vi "Simulation with Fixed-Point Inputs.vi"() -> ()   [LabVIEW 2023]
doc: "Demonstrates how to simulate the behavior of a fixed-point filter with actual fixed-point inputs."
uses:
  <vilib>/addons/Digital Filter Design/FXPModel.llb/DFD FXP Quantize Coef (Easy).vi
  <vilib>/Utility/VariantDataType/GetNumericFxpInfo.vi
  <vilib>/addons/Digital Filter Design/FXPSim.llb/dfd_Check Input FXP Settings.vi
  <vilib>/addons/Digital Filter Design/FXPSim.llb/dfd_Check SRate Simulation Integer Input.vi
  <vilib>/addons/Digital Filter Design/FXPSim.llb/dfd_FXP Simu.vi
  <vilib>/addons/Digital Filter Design/FXPSim.llb/DFD FXP Postprocessing (I32, 1Ch).vi
  <vilib>/addons/Digital Filter Design/_Objects.llb/DFD Quantization Sources.ctl
  <vilib>/addons/Digital Filter Design/_Objects.llb/DFD FXP Statistics Data.ctl
  <vilib>/addons/Digital Filter Design/FXPSim.llb/SimXnode/DFD FXP Simulation.xnode
  <vilib>/addons/Digital Filter Design/_Objects.llb/DFD Filter Obj.ctl
  <vilib>/addons/Digital Filter Design/_Objects.llb/DFD Filter Coef.ctl
  <vilib>/addons/Digital Filter Design/_Objects.llb/DFD Filter Structure Type Selector.ctl
  <vilib>/addons/Digital Filter Design/_Objects.llb/dfd_Internal Quantization Settings.ctl
  <vilib>/addons/Digital Filter Design/_Objects.llb/dfd_Internal Quantization Srcs.ctl
  <vilib>/addons/Digital Filter Design/_Objects.llb/DFD Coef Norm Type.ctl
  <vilib>/addons/Digital Filter Design/NI_DigFilterLicensed.lvlib
  <vilib>/Analysis/NI_AALBase.lvlib
  <vilib>/addons/Digital Filter Design/NI_DigFilter_FXP.lvlib
  <vilib>/Utility/VariantDataType/VariantType.lvlib
panel:
  out "Filtering Text Report":string
  in  "Output Word Length":i16=16
  out "Error Message":string
  out "Filtering Results":dbl[](graph)
  # "Select Help>>Show Context Help and move the cursor over the VI icon for more information."
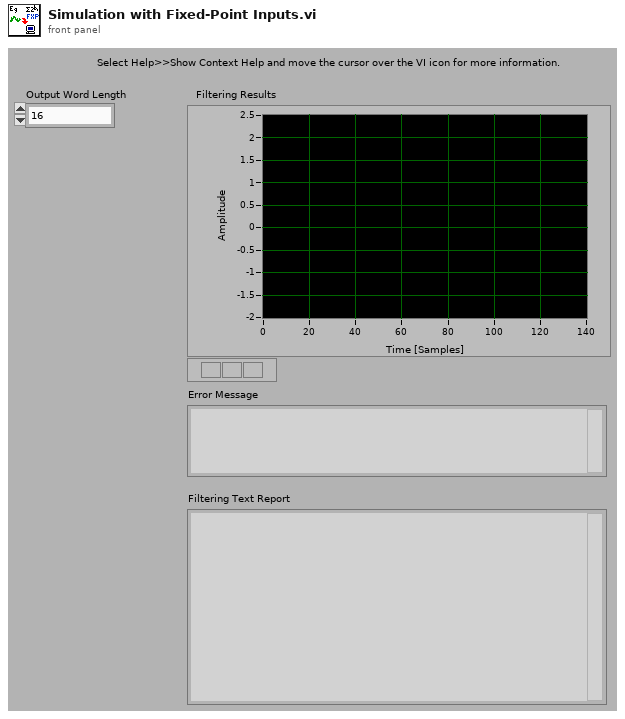
[diagram p1: front panel]
types:
  T1 = enum16{"Butterworth", "Chebyshev", "Inverse Chebyshev", "Elliptic", "Kaiser Window", "Dolph-Chebyshev Window", "Equi-Ripple FIR"}
  T2 = typedef "NI_DigFilterLicensed.lvlib/DFD Filter Obj.ctl" = cluster{"mSRate_Fs":dbl, "mSRate_Version":string, "mSRate_Comments":string, "mSRate_OrgCoef":T3, "mSRate_CurCoef":T3, "mSRate_Quantized?":bool, "mSRate_QCoef":T3, "mSRate_QSettings":T5[], "mSRate_Order":i32, "mSRate_Scaling":cluster{"mSRate_ScaleByPowerOf2?":bool, "mSRate_ScaleType":T7}}
  T3 = typedef "NI_DigFilterLicensed.lvlib/DFD Filter Coef.ctl" = cluster{"type":T4, "gain":dbl, "coef a (k)":dbl[], "coef b (v)":dbl[]}
  T4 = typedef "NI_DigFilterLicensed.lvlib/DFD Filter Structure Type Selector.ctl" = enum16{"Undefined", "FIR Direct Form", "FIR Direct Form Transposed", "FIR Symmetric", "FIR Antisymmetric", "IIR Direct Form I", "IIR Direct Form I Transposed", "IIR Direct Form II", "IIR Direct Form II Transposed", "IIR Cascaded Second Order Sections Form I", "IIR Cascaded Second Order Sections Form I Transposed", "IIR Cascaded Second Order Sections Form II", "IIR Cascaded Second Order Sections Form II Transposed", "Lattice Allpass (basic sections)", "Lattice Allpass (one multiplier sections)", "Lattice Allpass (normalized sections)", "Lattice AR (basic sections)", "Lattice AR (one multiplier sections)", "Lattice AR (normalized sections)", "Lattice MA (minimum phase)", "Lattice MA (maximum phase)", "Lattice ARMA (basic sections)", "Lattice ARMA (one multiplier sections)", "Lattice ARMA (normalized sections)"}
  T5 = typedef "NI_DigFilterLicensed.lvlib/dfd_Internal Quantization Settings.ctl" = cluster{"source":T6, "wl":i16, "iwl":i16, "overflow mode":enum16{"Saturation", "Wrap"}, "rounding mode":enum16{"Nearest", "Truncation"}, "signed?":bool}
  T6 = typedef "NI_DigFilterLicensed.lvlib/dfd_Internal Quantization Srcs.ctl" = u16
  T7 = typedef "NI_DigFilterLicensed.lvlib/DFD Coef Norm Type.ctl" = enum16{"No Norm", "Time Domain 1-Norm", "Time Domain 2-Norm", "Time Domain Inf-Norm"}
  T8 = typedef "NI_DigFilterLicensed.lvlib/DFD Quantization Sources.ctl" = u16
  T9 = typedef "NI_DigFilterLicensed.lvlib/DFD FXP Statistics Data.ctl" = cluster{"max value":ext, "min value":ext, "#overflows":i32, "#underflows":i32, "#operations":i32}
  T10 = cluster{"quantizer source":T8, "statistics information":T9}[]
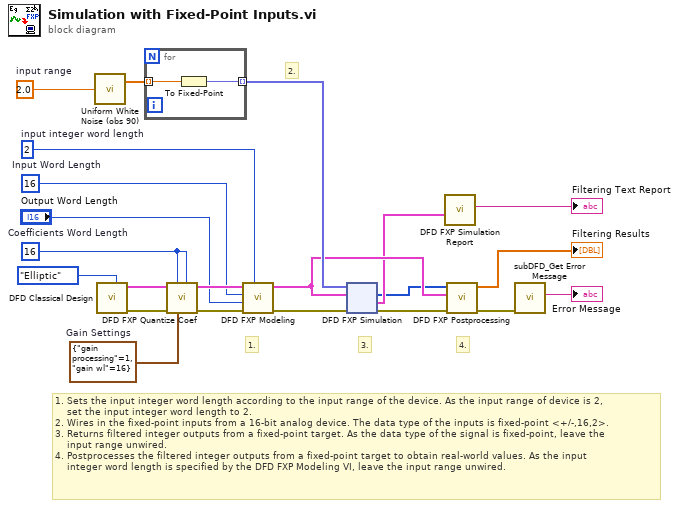
[diagram p0: block diagram]
diagram:
  w11 = i16 2  # input integer word length
  w13 = 2.0  # input range
  w12 = i16 16  # Input Word Length
  w18 = cluster{"gain processing":u16, "gain wl":i16} {"gain processing"=1, "gain wl"=16}  # Gain Settings
  w19 = i16 16  # Coefficients Word Length
  # "3."
  # "4."
  # "2."
  # "1."
  # "1. Sets the input integer word length according to the input range of the device. As the input range of device is 2,\n    set the input integer word length to 2.\n2. Wires in the fixed-point inputs from a 16-bit analog device. The data type of the inputs is fixed-point <+/-,16,2>.\n3. Returns filtered integer outputs from a fixed-point target. As the data type of the signal is fixed-point, leave the \n    input range unwired. \n4. Postprocesses the filtered integer outputs from a fixed-point target to obtain real-world values. As the input \n    integer word length is specified by the DFD FXP Modeling VI, leave the input range unwired."
  n1 = call <vilib>:"Uniform White Noise (obs 90).vi"("amplitude"=w13) -> ("uniform white noise"=w8:dbl[])  [unwired: 2 in, 1 out]
  n2 = call <vilib>:"DFD Classical Design.vi"("design method"=T1."Elliptic") -> ("error out"=w20:errorcluster, "filter out"=w10:T2)  [unwired: 5 in, 4 out]
  n3 = for {
    tunnel: w8 -> [w24] mode=indexing
    tunnel: [w23] -> w6 mode=indexing
    n4 = To Fixed-Point(number=w24) -> (fixed-point=w23:fxp<+/-,16,2>)  [unwired: 1 out]
  }
  n5 = call-poly <vilib>:"DFD FXP Quantize Coef.vi"("coefficients b/v word length"=w19, "gain settings"=w18, "coefficients a/k word length"=w19, "error in (no error)"=w20, "filter in"=w10) -> ("error out"=w16:errorcluster, "filter out"=w17:T2)  [unwired: 5 out]
  n6 = call <vilib>:"DFD FXP Modeling.vi"("input integer word length"=w11, "error in (no error)"=w16, "output word length"="Output Word Length", "input word length"=w12, "filter in"=w17) -> ("error out"=w4:errorcluster, "filter out"=w5:T2)  [unwired: 2 in, 3 out]
  n7 = xnode "DFD FXP Simulation"("error in (no error)"=w4, "filter in"=w5, "signal in"=w6) -> ("error out"=w3:errorcluster, "filtering statistics report"=w2:T10, "integer signal out"=w1:i32[])  [unwired: 3 in, 1 out]
  n8 = call <vilib>:"DFD FXP Simulation Report.vi"("filtering statistics report"=w2) -> ("filtering text report"=→"Filtering Text Report":string)  [unwired: 1 in, 9 out]
  n9 = call-poly <vilib>:"DFD FXP Postprocessing.vi"("error in (no error)"=w3, "filter"=w5, "signal in"=w1) -> ("error out"=w14:errorcluster, "signal out"=→"Filtering Results":dbl[])  [unwired: 1 in, 6 out]
  n10 = call <vilib>:"subDFD_Get Error Message.vi"("error in (no error)"=w14) -> ("Error Message"=→"Error Message":string)  [unwired: 10 out]
